vi "Iterate.vi"(8 "error in (no error)":errorcluster, 11 "Object ref in":T1) -> (0 "error out":errorcluster, 2 "Finished?":bool, 3 "Object ref out":T1, 4 "Current iteration":i32, 6 "Current layer":i32)   [LabVIEW 2013, in "SLMControl.lvlib" / "SC-Main.lvclass"]
uses:
  SC-Main.lvclass
  Object-reference.ctl
  SC-Main.lvclass/SC-Main.ctl
  Vision-actions.ctl
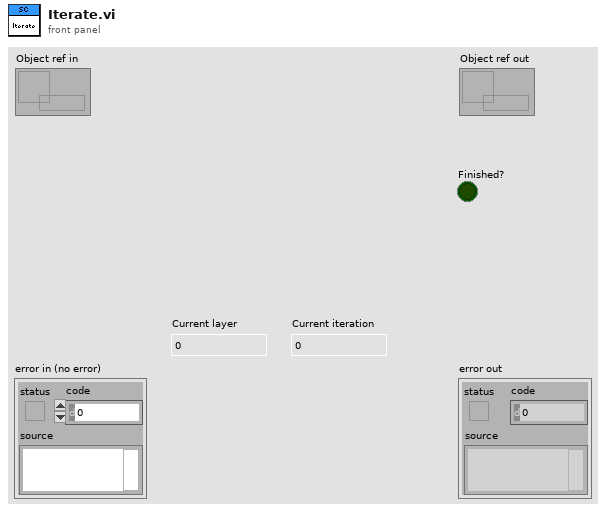
[diagram p1: front panel]
types:
  T1 = typedef "SLMControl.lvlib/SC-Main.lvclass/Object-reference.ctl" = refnum<data-value>
  T2 = typedef "SLMControl.lvlib/SC-Main.lvclass/Vision-actions.ctl" = enum16{"Activate", "Start", "Repeat", "Stop", "Exit"}
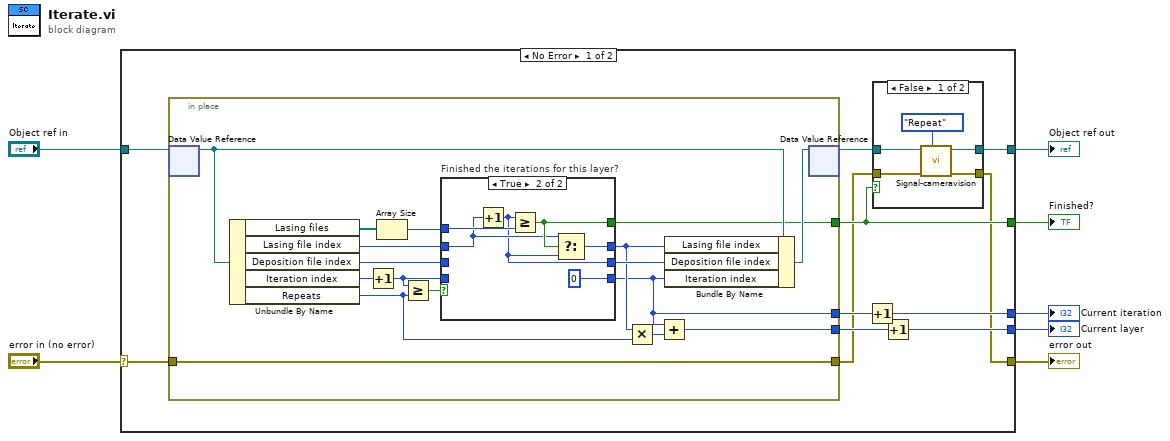
[diagram p0: block diagram]
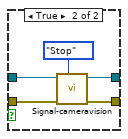
[diagram p2: hidden frame]
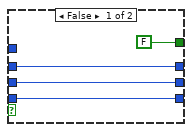
[diagram p3: hidden frame]
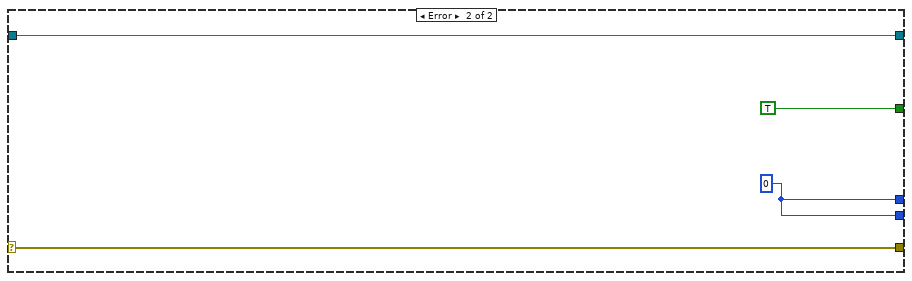
[diagram p4: hidden frame]
diagram:
  n1 = case shown="No Error" "error in (no error)" {
    selector: "error in (no error)" -> [w18 w59]
    tunnel: [w8 w59] -> w6
    tunnel: [w10 w58] -> w4
    tunnel: "Object ref in" -> [w17 w58]
    tunnel: [w12 TRUE] -> w3
    tunnel: [w15 w56] -> w2
    tunnel: [w13 w56] -> w1
    frame No Error {
      n2 = in-place {
        in-place-border: w18 -> [w36]
        in-place-border: [w36] -> w9
        in-place-border: [w34] -> w12
        in-place-border: [w30] -> w16
        in-place-border: [w29] -> w14
        n3 = in-place-dvr #1(w17) -> (w38:refnum<class "SC-Main.lvclass">)  [unwired: 1 out]
        n4 = Unbundle By Name(w38) -> ("Lasing files"=w45:path[], "Lasing file index"=w44:i32, "Deposition file index"=w43:i32, "Iteration index"=w42:i32, "Repeats"=w31:i32)
        n5 = Increment(x=w42) -> (x+1=w35:i32)
        n6 = Array Size(array=w45) -> (size(s)=w40:i32)
        n7 = Greater Or Equal?(x=w35, y=w31) -> (x >= y?=w41:bool)
        n8 = case "Finished the iterations for this layer?" shown="True" w41 {
          tunnel: w44 -> [w48 w51]
          tunnel: w43 -> [w47 _]
          tunnel: w40 -> [_ w55]
          tunnel: [FALSE w53] -> w34
          tunnel: [w48 w52] -> w32
          tunnel: [w47 w50] -> w39
          tunnel: w35 -> [w49 _]
          tunnel: [w49 0] -> w30
          frame False {
          }
          frame True {
            n9 = Increment(x=w51) -> (x+1=w50:i32)
            n10 = Greater Or Equal?(x=w50, y=w55) -> (x >= y?=w53:bool)
            n11 = Select(t=w51, s=w53, f=w50) -> (s? t:f=w52:i32)
          }
        }
        n12 = Multiply(x=w32, y=w31) -> (x*y=w33:i32)
        n13 = Add(x=w30, y=w33) -> (x+y=w29:i32)
        n14 = Bundle By Name(cluster=w38, "Lasing file index"=w32, "Deposition file index"=w39, "Iteration index"=w30) -> (w37:refnum<class "SC-Main.lvclass">)
        n15 = in-place-dvr #1(w37) -> (w11:T1)  [unwired: 1 out]
      }
      n16 = Increment(x=w16) -> (x+1=w15:i32)
      n17 = case shown="False" w12 {
        tunnel: w11 -> [w22 w27]
        tunnel: [w19 w26] -> w10
        tunnel: w9 -> [w21 w25]
        tunnel: [w20 w24] -> w8
        frame False {
          n18 = call "Signal-cameravision.vi"("Vision action"=Vision-actions."Repeat", "error in (no error)"=w21, "Object ref in"=w22) -> ("error out"=w20:errorcluster, "Object ref out"=w19:T1)  [unwired: 7 in]
        }
        frame True {
          n19 = call "Signal-cameravision.vi"("Vision action"=Vision-actions."Stop", "error in (no error)"=w25, "Object ref in"=w27) -> ("error out"=w24:errorcluster, "Object ref out"=w26:T1)  [unwired: 7 in]
        }
      }
      n20 = Increment(x=w14) -> (x+1=w13:i32)
    }
    frame Error {
      w56 = 0
    }
  }
  "error out" <- w6
  "Object ref out" <- w4
  "Current layer" <- w1
  "Current iteration" <- w2
  "Finished?" <- w3
